vi "PH_SHS_Analysis.panel.vi"(0 "object ref":refnum<vi>, 5 "error in (no error)":errorcluster) -> (19 "error out":errorcluster)   [LabVIEW 2014, in "PH_SHS_Analysis.lvlib"]
doc: "This a GUI.\n\nLicense Agreement for this software:\n\nCopyright (C)\nGesellschaft für Schwerionenforschung, GSI\nPlanckstr. 1\n64291 Darmstadt\nGermany\n\nContact: D.Beck@gsi.de \n\nThis program is free software; you can redistribute it and/or modify it under the terms of the GNU General Public License as published by the Free Software Foundation; either version 2 of the license, or (at your option) any later version.\n\nThis program is distributed in the hope that it will be useful, but WITHOUT ANYW ARRANTY; without even the implied warranty of MERCHANTABILITY or FITNESS FOR A PARTICULAR PURPOSE. See the GNU General License for more details (http://www.gnu.org).\n\nGesellschaft für Schwerionenforschung, GSI\nPlanckstr. 1, 64291 Darmstadt, Germany\nFor all questions and ideas contact: M.Richter@gsi.de, H.Brand@gsi.de or D.Beck@gsi.de.\nLast update: 18-DEC-2002"
uses:
  PH_SHS_Analysis.lvlib
  PH_SHS_Analysis_Calibrator/PH_SHS_Analysis_Calibrator.Analysis Calibration Data.ctl
  User/Eisenbarth/SHS_v4/SHS_Common/SHSReference.ctl
  User/Eisenbarth/SHS_v4/SHS_Common/ReferencePoint.ctl
  User/Eisenbarth/SHS_v4/SHS_Common/Rectangle.ctl
  User/Eisenbarth/SHS_v4/SHS_Common/Point.ctl
  PH_SHS_Analysis.Result.ctl
  PH_SHS_Analysis.Zernike Coefficients.ctl
  User/Eisenbarth/SHS_v4/SHS_Common/Shifts.ctl
  PH_Img_BaseClass/PH_Img_BaseClass.Palette.ctl
  PH_Img_BaseClass/PH_Img_BaseClass.GUI Refs.ctl
  CSCore/CSObj/CSObj.lvlib
  PH_Common/PH_Common.lvlib
  CSCore/CSSystem/CSSystemLib/CSSystemLib.lvlib
  PH_Img_BaseClass/PH_Img_BaseClass.lvlib
  PH_Class/PH_Class.lvlib
  PH_PSDBWriter/PH_PSDBWriter.lvlib
  User/Eisenbarth/SHS_v4/SHS_Common/SHS_Common.lvlib
  PH_SHS_Analysis_Calibrator/PH_SHS_Analysis_Calibrator.lvlib
panel:
  out "Publishing Data Status":u32(colorbox)=16860 caption="Status"
  out "Calibration status":u32(colorbox)=16860 caption="Calibration"
  out "Timeout":u32(colorbox)=16860
  in  "Tab Control":T1(tab)
  in  "Take Cali \nReference":bool caption="On"
  in  "Remove Tilt":bool caption="On"
  in  "Consider Tilt":bool caption="On"
  out "Result":T2 {"Measurement Quality" scale=0.0..12.0; "Zernike Coefficients"."2nd Spherical" scale=-2.0..2.0 scale format="%.2f"; "Zernike Coefficients"."2nd Coma y" scale=-2.0..2.0 scale format="%.2f"; "Zernike Coefficients"."2nd Coma x" scale=-2.0..2.0 scale format="%.2f"; "Zernike Coefficients"."2nd Astig 45°" scale=-2.0..2.0 scale format="%.2f"; "Zernike Coefficients"."2nd Astig 0°" scale=-2.0..2.0 scale format="%.2f"; "Zernike Coefficients"."Trefoil 30°" scale=-2.0..2.0 scale format="%.2f"; "Zernike Coefficients"."Trefoil 0°" scale=-2.0..2.0 scale format="%.2f"; "Zernike Coefficients"."Spherical" scale=-2.0..2.0 scale format="%.2f"; "Zernike Coefficients"."Coma y" scale=-2.0..2.0 scale format="%.2f"; "Zernike Coefficients"."Coma x" scale=-2.0..2.0 scale format="%.2f"; "Zernike Coefficients"."Astig 45°" scale=-2.0..2.0 scale format="%.2f"; "Zernike Coefficients"."Astig 0°" scale=-2.0..2.0 scale format="%.2f"; "Zernike Coefficients"."Defocus" scale=-2.0..2.0 scale format="%.2f"; "Zernike Coefficients"."Tilt y" scale=-2.0..2.0 scale format="%.2f"; "Zernike Coefficients"."Tilt x" scale=-2.0..2.0 scale format="%.2f"; "Time Stamp" format="%<%H:%M:%S%2u\n%y/%m/%d>T"}
  in  "Timeout Set":i32 caption="ms"
  in  "Global On":bool caption="On"
  in  "Palette":T6 items=["Grey", "Binary", "Gradient", "Rainbow", "Temperature"]
  in  "Show overlay":bool
  out "GUI Image":T7(plugin-control)
  in  "Calibration Data File":path
  out "SHS Analysis Calibration Data":T8
  out "Cam Source":string
  in  "SHS Device Config":T12={"focal length [m]"=0.01, "pixel size [m/px]"=6.7e-06, "wavelength [m]"=1.053e-06} {"wavelength [m]" format="%#_6p"; "pixel size [m/px]" format="%#_6p"; "focal length [m]" format="%#_6p"}
  out "Working Reference":T13
  out "PSDB Status":u32(colorbox)=6618880 caption="PSDB"
  in  "Delete":bool
  in  "Exit":bool
  # "PCS"
  # "3.40"
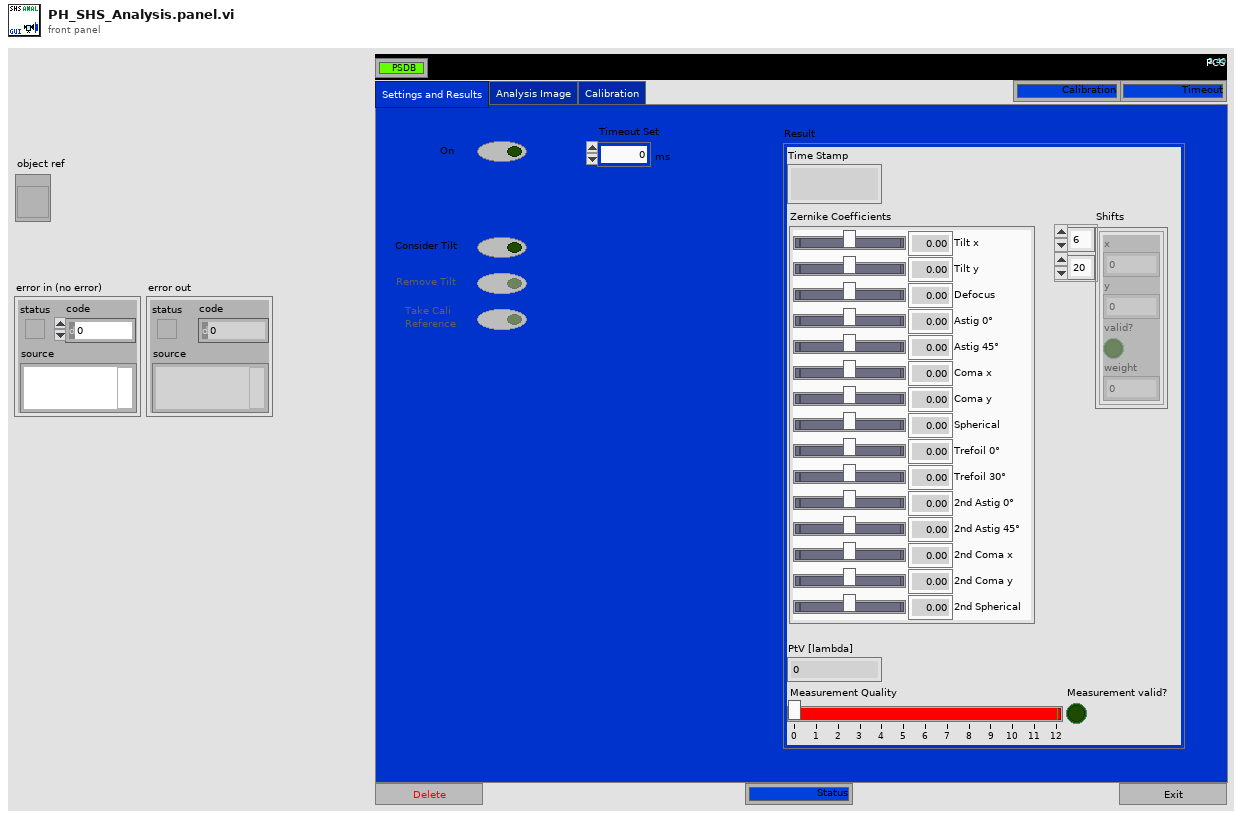
[diagram p1: front panel]
types:
  T1 = enum32{"Settings and Results", "Analysis Image", "Calibration"}
  T2 = typedef "PH_SHS_Analysis.lvlib/PH_SHS_Analysis.Result.ctl" = cluster{"Time Stamp":timestamp, "Zernike Coefficients":T3, "PtV [lambda]":dbl, "Shifts":T4, "Measurement Quality":cluster{dbl, dbl, dbl}, "Measurement valid?":bool}
  T3 = typedef "PH_SHS_Analysis.lvlib/PH_SHS_Analysis.Zernike Coefficients.ctl" = cluster{"Tilt x":dbl, "Tilt y":dbl, "Defocus":dbl, "Astig 0°":dbl, "Astig 45°":dbl, "Coma x":dbl, "Coma y":dbl, "Spherical":dbl, "Trefoil 0°":dbl, "Trefoil 30°":dbl, "2nd Astig 0°":dbl, "2nd Astig 45°":dbl, "2nd Coma x":dbl, "2nd Coma y":dbl, "2nd Spherical":dbl}
  T4 = typedef "SHS_Common.lvlib/Shifts.ctl" = T5[][]
  T5 = typedef "SHS_Common.lvlib/Point.ctl" = cluster{"x":dbl, "y":dbl, "valid?":bool, "weight":dbl}
  T6 = typedef "PH_Img_BaseClass.lvlib/PH_Img_BaseClass.Palette.ctl" = i32
  T7 = typedef "IMAQ Image.ctl" = refnum<image>
  T8 = typedef "PH_SHS_Analysis_Calibrator.lvlib/PH_SHS_Analysis_Calibrator.Analysis Calibration Data.ctl" = cluster{"Date":string, "Time":string, "Cam Settings":cluster{"Cam ID":string, "Gain":dbl, "Brightness":dbl, "Shutter":dbl, "Cam Error":bool, "Mode":i32}, "SHS Reference Result":T9, "Pixel Size":dbl, "MLA Pitch":dbl, "Method":enum16{"automatic", "manual"}, "Calibration Data calculated":bool, "No Problems at calculation?":bool, "error out":errorcluster}
  T9 = typedef "SHS_Common.lvlib/SHSReference.ctl" = cluster{"Reference":T10[][], "Lens Array Pitch [px]":dbl}
  T10 = typedef "SHS_Common.lvlib/ReferencePoint.ctl" = cluster{"Rect":T11, "Point":T5}
  T11 = typedef "SHS_Common.lvlib/Rectangle.ctl" = cluster{"Left":i32, "Top":i32, "Right":i32, "Bottom":i32}
  T12 = cluster{"focal length [m]":dbl, "pixel size [m/px]":dbl, "wavelength [m]":dbl}
  T13 = cluster{"Reference":T10[][], "Lens Array Pitch [px]":dbl}
  T14 = typedef "PH_Img_BaseClass.lvlib/PH_Img_BaseClass.GUI Refs.ctl" = cluster{"Timeout":refnum<vi>, "Image":refnum<vi>, "Palette":refnum<vi>, "Timeout Set":refnum<vi>}
  T15 = typedef "PH_SHS_Analysis.lvlib/PH_SHS_Analysis.i attribute.ctl" = cluster{"GUI Refs":cluster{"Delete":refnum<vi>, "Global On":refnum<vi>, "Cam Source":refnum<vi>, "Calibration Data File":refnum<vi>, "Calibration status":refnum<vi>, "Show overlay":refnum<vi>, "SHS Device Config":refnum<vi>, "Result":refnum<vi>, "Consider Tilt":refnum<vi>, "Working Reference":refnum<vi>, "Remove Tilt":refnum<vi>, "Take Cali  Reference":refnum<vi>, "Publishing Data Status":refnum<vi>, "Calibration Data":refnum<vi>}, "Calibration":cluster{"Status":T16, "Data":T8, "File":path}, "Result":T2, "Image":T7, "SHS Device Config":T17, "Show Overlay":bool, "GradientZernikeMatrix":dbl[][], "Consider Tilt":bool, "Working Reference":T9, "Zernicke Service ID":i32, "PSDB Image":T7}
  T16 = typedef "PH_StatusHandler.lvlib/PH_StatusHandler.Status.ctl" = i16
  T17 = typedef "SHS_Analysis.lvlib/SHS_DeviceConfig.ctl" = cluster{"focal length [m]":dbl, "pixel size [m/px]":dbl, "wavelength [m]":dbl}
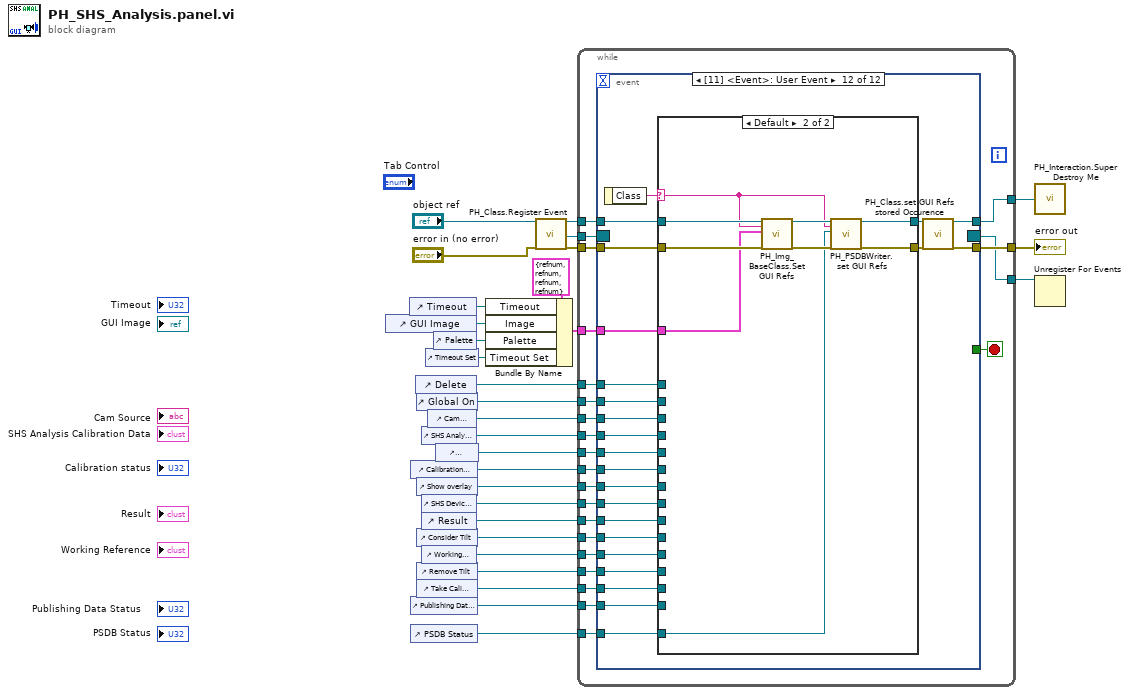
[diagram p0: block diagram]
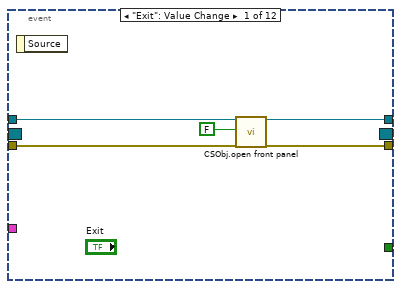
[diagram p2: hidden frame]
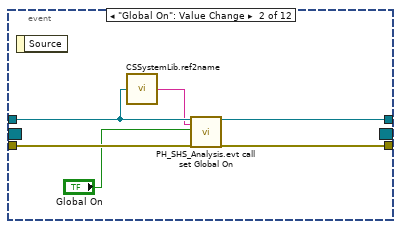
[diagram p3: hidden frame]
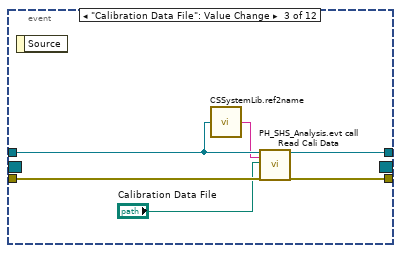
[diagram p4: hidden frame]
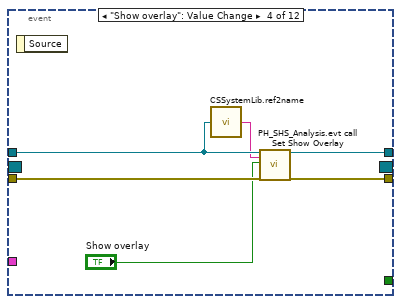
[diagram p5: hidden frame]
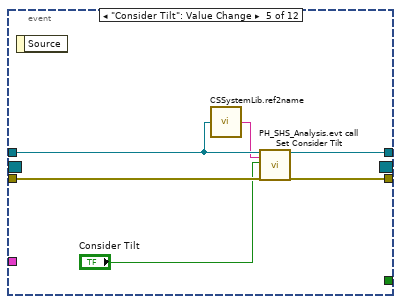
[diagram p6: hidden frame]
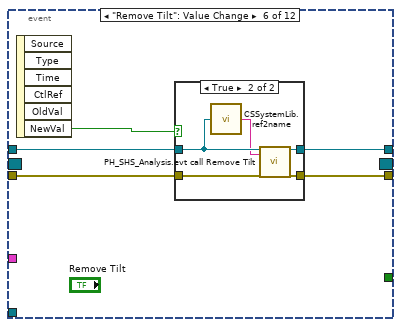
[diagram p7: hidden frame]
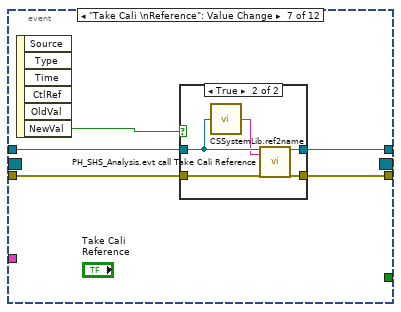
[diagram p9: hidden frame]
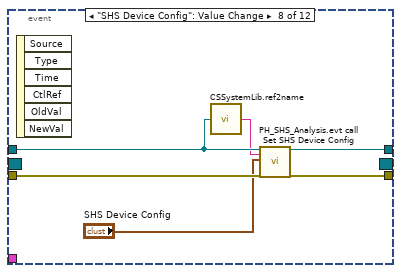
[diagram p11: hidden frame]
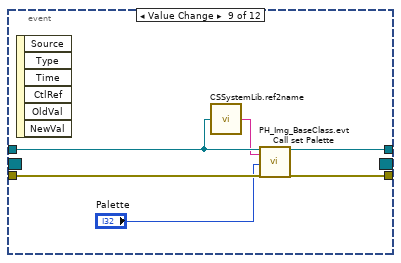
[diagram p12: hidden frame]
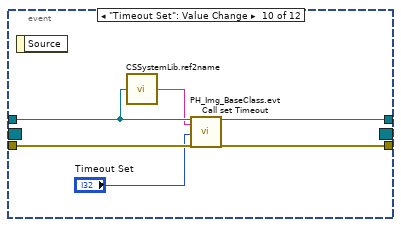
[diagram p13: hidden frame]
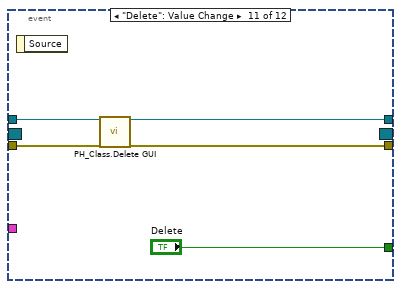
[diagram p14: hidden frame]
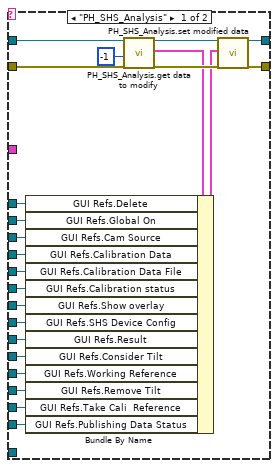
[diagram p15: hidden frame]
diagram:
  n1 = control-ref of="GUI Image"() -> (w25:refnum<vi>)
  n2 = control-ref of="Timeout"() -> (w26:refnum<vi>)
  n3 = control-ref of="Calibration status"() -> (w9:refnum<vi>)
  n4 = control-ref of="Publishing Data Status"() -> (w1:refnum<vi>)
  n5 = control-ref of="PSDB Status"() -> (w17:refnum<vi>)
  n6 = control-ref of="Delete"() -> (w14:refnum<vi>)
  n7 = control-ref of="Global On"() -> (w13:refnum<vi>)
  n8 = control-ref of="Show overlay"() -> (w8:refnum<vi>)
  n9 = control-ref of="Consider Tilt"() -> (w5:refnum<vi>)
  n10 = control-ref of="Remove Tilt"() -> (w3:refnum<vi>)
  n11 = control-ref of="Take Cali \nReference"() -> (w2:refnum<vi>)
  n12 = control-ref of="SHS Analysis Calibration Data"() -> (w11:refnum<vi>)
  n13 = control-ref of="SHS Device Config"() -> (w7:refnum<vi>)
  n14 = control-ref of="Result"() -> (w6:refnum<vi>)
  n15 = control-ref of="Working Reference"() -> (w4:refnum<vi>)
  n16 = control-ref of="Timeout Set"() -> (w23:refnum<vi>)
  n17 = control-ref of="Cam Source"() -> (w12:refnum<vi>)
  n18 = control-ref of="Palette"() -> (w24:refnum<vi>)
  n19 = control-ref of="Calibration Data File"() -> (w10:refnum<vi>)
  n20 = Bundle By Name(cluster=T14 {"Timeout"=refnum, "Image"=refnum, "Palette"=refnum, "Timeout Set"=refnum} ("GUI Refs"), "Timeout"=w26, "Image"=w25, "Palette"=w24, "Timeout Set"=w23) -> (w18:T14)
  n21 = call "PH_Class.Register Event.vi"("i ref in"="object ref", "error in (no error)"="error in (no error)") -> ("i ref out"=w22:refnum<vi>, "Event Registration Refnum"=w20:refnum<event-registration>, "error out"=w21:errorcluster)  [unwired: 15 in]
  n22 = while {
    tunnel: w22 -> [w49]
    tunnel: [w48] -> w29
    tunnel: w21 -> [w51]
    tunnel: [w50] -> w28
    tunnel: w20 -> [w47]
    tunnel: [w46] -> w19
    tunnel: w18 -> [w45]
    tunnel: w17 -> [w44]
    tunnel: w14 -> [w43]
    tunnel: w13 -> [w42]
    tunnel: w12 -> [w41]
    tunnel: w11 -> [w40]
    tunnel: w10 -> [w39]
    tunnel: w9 -> [w38]
    tunnel: w8 -> [w37]
    tunnel: w7 -> [w36]
    tunnel: w6 -> [w35]
    tunnel: w5 -> [w34]
    tunnel: w4 -> [w33]
    tunnel: w3 -> [w32]
    tunnel: w2 -> [w31]
    tunnel: w1 -> [w30]
    stop <- w52 stop-if-true
    n23 = event shown="[11] <Event>: User Event" {
      selector: w47 -> [_ _ _ _ _ _ _ _ _ _ _ _]
      dyn-events: [_ _ _ _ _ _ _ _ _ _ _ _] -> w46
      timeout: _ -> [_ _ _ _ _ _ _ _ _ _ _ _]
      tunnel: [_ _ _ _ _ _ _ _ _ _ "Delete" _] -> w52
      tunnel: w49 -> [w54 w59 w67 w73 w79 w84 w96 w109 w115 w120 w127 w151]
      tunnel: w51 -> [w57 w63 w69 w75 w81 w86 w98 w111 w117 w123 w126 w150]
      tunnel: [w56 w62 w68 w74 w80 w85 w97 w110 w116 w122 w124 w144] -> w50
      tunnel: [w53 w61 w66 w72 w78 w83 w95 w108 w114 w121 w125 w145] -> w48
      tunnel: w45 -> [_ _ _ _ _ _ _ _ _ _ _ w148]
      tunnel: w44 -> [_ _ _ _ _ _ _ _ _ _ _ w143]
      tunnel: w43 -> [_ _ _ _ _ _ _ _ _ _ _ w142]
      tunnel: w42 -> [_ _ _ _ _ _ _ _ _ _ _ w141]
      tunnel: w41 -> [_ _ _ _ _ _ _ _ _ _ _ w140]
      tunnel: w40 -> [_ _ _ _ _ _ _ _ _ _ _ w139]
      tunnel: w39 -> [_ _ _ _ _ _ _ _ _ _ _ w138]
      tunnel: w38 -> [_ _ _ _ _ _ _ _ _ _ _ w137]
      tunnel: w37 -> [_ _ _ _ _ _ _ _ _ _ _ w136]
      tunnel: w36 -> [_ _ _ _ _ _ _ _ _ _ _ w135]
      tunnel: w35 -> [_ _ _ _ _ _ _ _ _ _ _ w134]
      tunnel: w34 -> [_ _ _ _ _ _ _ _ _ _ _ w133]
      tunnel: w33 -> [_ _ _ _ _ _ _ _ _ _ _ w132]
      tunnel: w32 -> [_ _ _ _ _ _ _ _ _ _ _ w131]
      tunnel: w31 -> [_ _ _ _ _ _ _ _ _ _ _ w130]
      tunnel: w30 -> [_ _ _ _ _ _ _ _ _ _ _ w129]
      event "Exit": Value Change {
        n24 = event-data() -> ()  [unwired: 1 in, 1 out]
        n25 = call "CSObj.open front panel.vi"("i ref in"=w54, "frontPanelOpen"=FALSE ("front panel open"), "error in (no error)"=w57) -> ("i ref out"=w53:refnum<vi>, "error out"=w56:errorcluster)  [unwired: 15 in]
      }
      event "Global On": Value Change {
        n26 = event-data() -> ()  [unwired: 1 in, 1 out]
        n27 = call "CSSystemLib.ref2name.vi"("obj refnum"=w59) -> ("name"=w58:string)
        n28 = call "PH_SHS_Analysis.evt call set Global On.vi"("i ref in"=w59, "Instance"=w58, "Global On"="Global On", "error in (no error)"=w63) -> ("i ref out"=w61:refnum<vi>, "error out"=w62:errorcluster)  [unwired: 14 in]
      }
      event "Calibration Data File": Value Change {
        n29 = event-data() -> ()  [unwired: 1 in, 1 out]
        n30 = call "CSSystemLib.ref2name.vi"("obj refnum"=w67) -> ("name"=w65:string)
        n31 = call "PH_SHS_Analysis.evt call Read Cali Data.vi"("i ref in"=w67, "Instance"=w65, "Cali Data File"="Calibration Data File", "error in (no error)"=w69) -> ("i ref out"=w66:refnum<vi>, "error out"=w68:errorcluster)  [unwired: 14 in]
      }
      event "Show overlay": Value Change {
        n32 = event-data() -> ()  [unwired: 1 in, 1 out]
        n33 = call "CSSystemLib.ref2name.vi"("obj refnum"=w73) -> ("name"=w71:string)
        n34 = call "PH_SHS_Analysis.evt call Set Show Overlay.vi"("i ref in"=w73, "Instance"=w71, "Show Overlay"="Show overlay", "error in (no error)"=w75) -> ("i ref out"=w72:refnum<vi>, "error out"=w74:errorcluster)  [unwired: 14 in]
      }
      event "Consider Tilt": Value Change {
        n35 = event-data() -> ()  [unwired: 1 in, 1 out]
        n36 = call "CSSystemLib.ref2name.vi"("obj refnum"=w79) -> ("name"=w77:string)
        n37 = call "PH_SHS_Analysis.evt call Set Consider Tilt.vi"("i ref in"=w79, "Instance"=w77, "Consider Tilt"="Consider Tilt", "error in (no error)"=w81) -> ("i ref out"=w78:refnum<vi>, "error out"=w80:errorcluster)  [unwired: 14 in]
      }
      event "Remove Tilt": Value Change {
        n38 = event-data() -> ("NewVal"=w82:bool)  [unwired: 1 in, 5 out]
        n39 = case shown="True" w82 {
          tunnel: w86 -> [w87 w93]
          tunnel: [w87 w92] -> w85
          tunnel: w84 -> [w88 w91]
          tunnel: [w88 w90] -> w83
          frame False {
          }
          frame True {
            n40 = call "CSSystemLib.ref2name.vi"("obj refnum"=w91) -> ("name"=w89:string)
            n41 = call "PH_SHS_Analysis.evt call Remove Tilt.vi"("i ref in"=w91, "Instance"=w89, "error in (no error)"=w93) -> ("i ref out"=w90:refnum<vi>, "error out"=w92:errorcluster)  [unwired: 15 in]
          }
        }
      }
      event "Take Cali \nReference": Value Change {
        n42 = event-data() -> ("NewVal"=w94:bool)  [unwired: 1 in, 5 out]
        n43 = case shown="True" w94 {
          tunnel: w98 -> [w99 w105]
          tunnel: [w99 w104] -> w97
          tunnel: w96 -> [w100 w103]
          tunnel: [w100 w102] -> w95
          frame False {
          }
          frame True {
            n44 = call "CSSystemLib.ref2name.vi"("obj refnum"=w103) -> ("name"=w101:string)
            n45 = call "PH_SHS_Analysis.evt call Take Cali Reference.vi"("i ref in"=w103, "Instance"=w101, "error in (no error)"=w105) -> ("i ref out"=w102:refnum<vi>, "error out"=w104:errorcluster)  [unwired: 15 in]
          }
        }
      }
      event "SHS Device Config": Value Change {
        n46 = event-data() -> ()  [unwired: 1 in, 6 out]
        n47 = call "CSSystemLib.ref2name.vi"("obj refnum"=w109) -> ("name"=w107:string)
        n48 = call "PH_SHS_Analysis.evt call Set SHS Device Config.vi"("i ref in"=w109, "Instance"=w107, "SHS Device Config"="SHS Device Config", "error in (no error)"=w111) -> ("i ref out"=w108:refnum<vi>, "error out"=w110:errorcluster)  [unwired: 14 in]
      }
      event Value Change {
        n49 = event-data() -> ()  [unwired: 1 in, 6 out]
        n50 = call "CSSystemLib.ref2name.vi"("obj refnum"=w115) -> ("name"=w113:string)
        n51 = call "PH_Img_BaseClass.evt Call set Palette.vi"("i ref in"=w115, "Instance"=w113, "Palette"="Palette", "error in (no error)"=w117) -> ("i ref out"=w114:refnum<vi>, "error out"=w116:errorcluster)  [unwired: 14 in]
      }
      event "Timeout Set": Value Change {
        n52 = event-data() -> ()  [unwired: 1 in, 1 out]
        n53 = call "CSSystemLib.ref2name.vi"("obj refnum"=w120) -> ("name"=w119:string)
        n54 = call "PH_Img_BaseClass.evt Call set Timeout.vi"("i ref in"=w120, "Instance"=w119, "Timeout [ms]"="Timeout Set", "error in (no error)"=w123) -> ("i ref out"=w121:refnum<vi>, "error out"=w122:errorcluster)  [unwired: 14 in]
      }
      event "Delete": Value Change {
        n55 = event-data() -> ()  [unwired: 1 in, 1 out]
        n56 = call "PH_Class.Delete GUI.vi"("VI in"=w127, "error in (no error)"=w126) -> ("VI out"=w125:refnum<vi>, "error out"=w124:errorcluster)  [unwired: 16 in]
      }
      event User Event {
        n57 = event-data() -> ("Class"=w149:string)  [unwired: 1 in]
        n58 = case shown="Default" w149 {
          selector: w149 -> [_ w175]
          tunnel: w151 -> [w171 w183]
          tunnel: w150 -> [w170 w182]
          tunnel: [w169 w179] -> w146
          tunnel: [w168 w177] -> w147
          tunnel: w148 -> [_ w181]
          tunnel: w143 -> [_ w176]
          tunnel: w142 -> [w165 _]
          tunnel: w141 -> [w164 _]
          tunnel: w140 -> [w163 _]
          tunnel: w139 -> [w162 _]
          tunnel: w138 -> [w161 _]
          tunnel: w137 -> [w160 _]
          tunnel: w136 -> [w159 _]
          tunnel: w135 -> [w158 _]
          tunnel: w134 -> [w157 _]
          tunnel: w133 -> [w156 _]
          tunnel: w132 -> [w155 _]
          tunnel: w131 -> [w154 _]
          tunnel: w130 -> [w153 _]
          tunnel: w129 -> [w152 _]
          frame "PH_SHS_Analysis" {
            n59 = call "PH_SHS_Analysis.get data to modify.vi"("i ref in"=w171, "ms timeout (10000)"=-1, "error in (no error)"=w170) -> ("i ref out"=w172:refnum<vi>, "i attribute"=w166:T15, "error out"=w173:errorcluster)  [unwired: 13 in, 1 out]
            n60 = Bundle By Name(cluster=w166, "GUI Refs.Delete"=w165, "GUI Refs.Global On"=w164, "GUI Refs.Cam Source"=w163, "GUI Refs.Calibration Data"=w162, "GUI Refs.Calibration Data File"=w161, "GUI Refs.Calibration status"=w160, "GUI Refs.Show overlay"=w159, "GUI Refs.SHS Device Config"=w158, "GUI Refs.Result"=w157, "GUI Refs.Consider Tilt"=w156, "GUI Refs.Working Reference"=w155, "GUI Refs.Remove Tilt"=w154, "GUI Refs.Take Cali  Reference"=w153, "GUI Refs.Publishing Data Status"=w152) -> (w167:T15)
            n61 = call "PH_SHS_Analysis.set modified data.vi"("i ref in"=w172, "i attribute"=w167, "error in (no error)"=w173) -> ("i ref out"=w169:refnum<vi>, "error out"=w168:errorcluster)  [unwired: 15 in]
          }
          frame Default {
            n62 = call "PH_Img_BaseClass.Set GUI Refs.vi"("i ref in"=w183, "Class"=w175, "GUI Refs"=w181, "error in (no error)"=w182) -> ("i ref out"=w180:refnum<vi>, "error out"=w178:errorcluster)  [unwired: 14 in]
            n63 = call "PH_PSDBWriter.set GUI Refs.vi"("i ref in"=w180, "Class"=w175, "Ref PSDB Status"=w176, "error in"=w178) -> ("i ref out"=w179:refnum<vi>, "error out"=w177:errorcluster)  [unwired: 14 in]
          }
        }
        n64 = call "PH_Class.set GUI Refs stored Occurence.vi"("i ref in"=w146, "error in (no error)"=w147) -> ("i ref out"=w145:refnum<vi>, "error out"=w144:errorcluster)  [unwired: 16 in]
      }
    }
  }
  "error out" <- w28
  n65 = call "PH_Interaction.Super Destroy Me.vi"("i ref out"=w29) -> ()
  n66 = Unregister For Events(event registration refnum=w19) -> ()  [unwired: 1 in, 1 out]
